vi "Launcher.vi"   [LabVIEW 2017, in "MVA Example.lvlib"]
uses:
  MVA Example.lvlib
  ExampleViewManager/ExampleViewManager.lvclass
  C:/Program Files (x86)/National Instruments/LabVIEW 2017/vi.lib/Composed Systems/MVA Framework/Framework/IViewManager/IViewManager/IViewManager.lvclass
  C:/Program Files (x86)/National Instruments/LabVIEW 2017/vi.lib/Composed Systems/MVA Framework/Framework/IViewable/IViewable/IViewable.lvclass
  <vilib>/Composed Systems/MVA Framework/Framework/IModel/IModel/IModel.lvclass
  <vilib>/Composed Systems/MVA Framework/Framework/IViewable/IViewable/View Position Enum.ctl
  BooleanView/BooleanView.lvclass
  ChartView/ChartView.lvclass
  ListboxView/ListboxView.lvclass
  SlideView/SlideView.lvclass
  ExampleViewModel/ExampleViewModel.lvclass
  C:/Program Files (x86)/National Instruments/LabVIEW 2017/vi.lib/Composed Systems/MVA Framework/Framework/IViewModel/IViewModel/IViewModel.lvclass
  C:/Program Files (x86)/National Instruments/LabVIEW 2017/vi.lib/ActorFramework/Actor/Actor.lvclass
  <vilib>/Composed Systems/MVA Framework/Framework/IMediator/IMediator/IMediator.lvclass
  <vilib>/Composed Systems/MVA Framework/Framework/IViewManager/IViewManager Messages/Launch Nested Views Msg/Launch Nested Views Msg.lvclass/Launch Nested Views Msg.ctl
  <vilib>/Composed Systems/MVA Framework/Framework/IViewManager/IViewManager/IViewManager.lvclass/IViewManager.ctl
  <vilib>/Composed Systems/MVA Framework/Framework/IViewModel/IViewModel/IViewModel.lvclass/IViewModel.ctl
  <vilib>/Composed Systems/MVA Framework/Framework/IViewable/IViewable Messages/Open Front Panel Msg/Open Front Panel Msg.lvclass/Open Front Panel Msg.ctl
  <vilib>/ActorFramework/Message Enqueuer/Message Enqueuer.lvclass/Message Enqueuer.ctl
  <vilib>/Composed Systems/MVA Framework/Framework/IViewManager/IViewManager Messages/Launch Nested Views Msg/Pack Launch Nested Views Msg.vi
  <vilib>/Composed Systems/MVA Framework/Framework/IViewManager/IViewManager/Write Startup Launch Nested Views Msg.vi
  <vilib>/ActorFramework/Message Enqueuer/Enqueue.vi
  <vilib>/Composed Systems/MVA Framework/ViewManager/QuadViewManager/QuadViewManager.lvclass
  <vilib>/Composed Systems/MVA Framework/Framework/IViewModel/IViewModel/IViewModel.lvclass
  <vilib>/Composed Systems/MVA Framework/Framework/IViewable/IViewable Messages/Open Front Panel Msg/Open Front Panel Msg.lvclass
  C:/Program Files (x86)/National Instruments/LabVIEW 2017/vi.lib/ActorFramework/Message/Message.lvclass
  <vilib>/ActorFramework/Message Priority Queue/Priority Enqueue.vi
  <vilib>/Composed Systems/MVA Framework/Framework/IViewManager/IViewManager Messages/Launch Nested Views Msg/Launch Nested Views Msg.lvclass
  <vilib>/Composed Systems/MVA Framework/Framework/IViewable/IApplicationStyle/IApplicationStyle.lvclass
  <vilib>/ActorFramework/Actor/Actor.lvclass
  <vilib>/Composed Systems/MVA Framework/Framework/IViewable/IViewable/IViewable.lvclass
  <vilib>/Composed Systems/MVA Framework/Framework/IViewManager/IViewManager/IViewManager.lvclass
types:
  T1 = typedef "IViewable.lvlib/IViewable.lvclass/View Position Enum.ctl" = enum16{"Centered", "Maximized", "Minimized", "Custom", "Unchanged"}
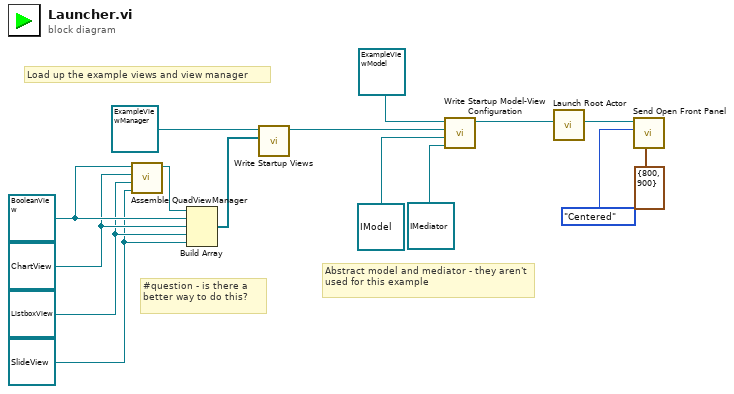
[diagram p0: block diagram]
diagram:
  w4 = refnum<class "SlideView.lvclass"> refnum ("MVA Example.lvlib:SlideView.lvclass")
  w5 = refnum<class "ListboxView.lvclass"> refnum ("MVA Example.lvlib:ListboxView.lvclass")
  w6 = refnum<class "ChartView.lvclass"> refnum ("MVA Example.lvlib:ChartView.lvclass")
  w7 = refnum<class "BooleanView.lvclass"> refnum ("MVA Example.lvlib:BooleanView.lvclass")
  # "Abstract model and mediator - they aren't used for this example"
  # "Load up the example views and view manager"
  # "#question - is there a better way to do this?"
  n1 = call <vilib>:"Assemble QuadViewManager.vi"("Bottom-Right View"=w4, "Bottom-Left View"=w5, "Top-Right View"=w6, "Top-Left View"=w7) -> ("QuadViewManager out"=w10:refnum<class "QuadViewManager.lvclass">)  [unwired: 7 in]
  n2 = Build Array(w10, w7, w6, w5, w4) -> (w11:refnum<class "IViewable.lvclass">[])
  n3 = call <vilib>:"Write Startup Views.vi"("Startup Views"=w11, "IViewManager in"=refnum<class "ExampleViewManager.lvclass"> refnum ("ExampleViewManager.lvlib:ExampleViewManager.lvclass")) -> ("IViewManager out"=w8:refnum<class "ExampleViewManager.lvclass">)  [unwired: 9 in]
  n4 = call <vilib>:"Write Startup Model-View Configuration.vi"("Mediator Type"=refnum<class "IMediator.lvclass"> refnum, "Model Type"=refnum<class "IModel.lvclass"> refnum, "Startup View Configuration"=w8, "IViewModel In"=refnum<class "ExampleViewModel.lvclass"> refnum ("MVA Example.lvlib:ExampleViewModel.lvclass")) -> ("IViewModel Out"=w15:refnum<class "ExampleViewModel.lvclass">)  [unwired: 7 in]
  n5 = call <vilib>:"Launch Root Actor.vi"("Actor"=w15) -> ("Actor's Enqueuer"=w14:refnum<class "Message Enqueuer.lvclass">)  [unwired: 9 in, 1 out]
  n6 = call <vilib>:"Send Open Front Panel.vi"("Custom Window Size"=cluster{"Height":i16, "Width":i16} {"Height"=800, "Width"=900}, "Position"=View_Position_Enum."Centered", "Message Enqueuer"=w14) -> ()  [unwired: 7 in, 2 out]
